vi "AI_ConfigurationRLC.vi"(8 "Error in":errorcluster, 10 "DAQ parameters":T1={"Trigger level"=1.0204081632653061, "Trigger slope"=10280, "Sampling rate (Hz)"=10000.0, "Number of sampes"=1000} {"Trigger slope" items=["Rising"=10280, "Falling"=10171]; "Trigger level" scale=0.0..10.0 scale format="%#_3g"}, 11 "Channels":T2) -> (0 "Error out":errorcluster, 3 "Task out":refnum<k21>)   [LabVIEW 2021]
uses:
  DAQmx_Channels.ctl
  DAQmx_Parameters.ctl
  <vilib>/DAQmx/create/channels.llb/DAQmx Create Channel (AI-Voltage-Basic).vi
  <vilib>/DAQmx/configure/timing.llb/DAQmx Timing (Sample Clock).vi
  <vilib>/DAQmx/configure/trigger.llb/DAQmx Start Trigger (Analog Edge).vi
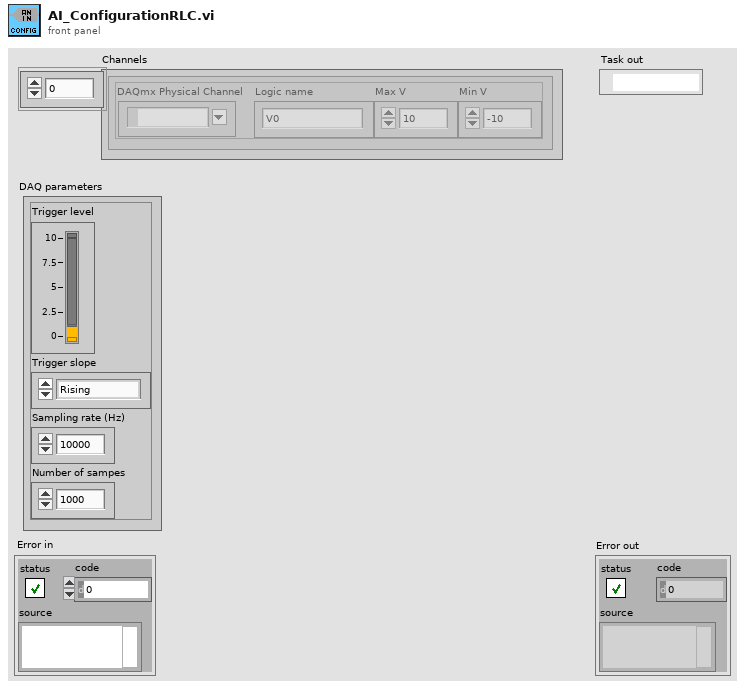
[diagram p1: front panel]
types:
  T1 = typedef "DAQmx_Parameters.ctl" = cluster{"Trigger level":dbl, "Trigger slope":u16, "Sampling rate (Hz)":dbl, "Number of sampes":i32}
  T2 = typedef "DAQmx_Channels.ctl" = cluster{"DAQmx Physical Channel":tag, "Logic name":string, "Max V":dbl, "Min V":dbl}[]
  T3 = cluster{"DAQmx Physical Channel":tag, "Logic name":string, "Max V":dbl, "Min V":dbl}
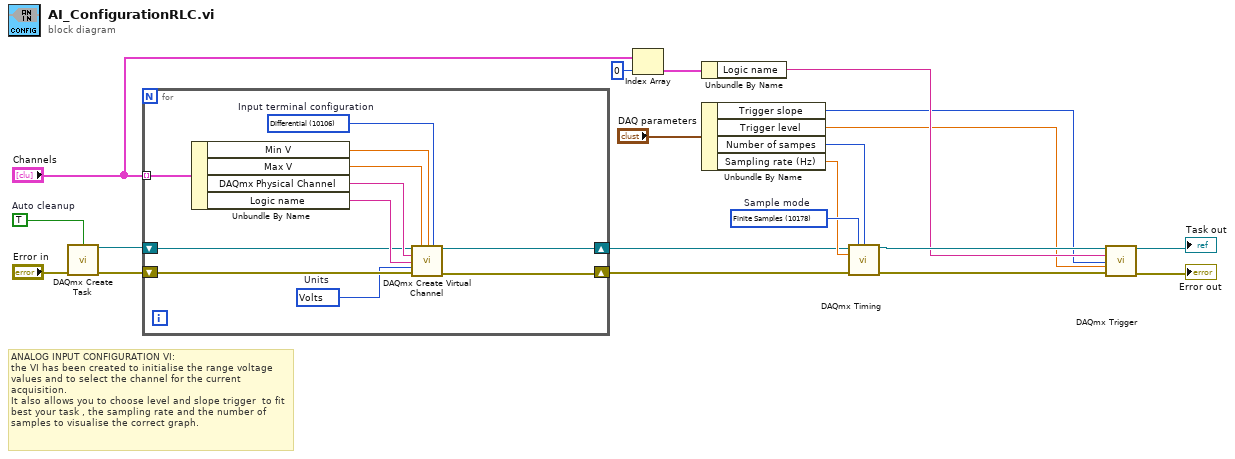
[diagram p0: block diagram]
diagram:
  w6 = TRUE  # Auto cleanup
  w17 = 10178 items=["Finite Samples"=10178, "Continuous Samples"=10123, "Hardware Timed Single Point"=12522]  # Sample mode
  # "ANALOG INPUT CONFIGURATION VI:\nthe VI has been created to initialise the range voltage values and to select the channel for the current acquisition. \nIt also allows you to choose level and slope trigger  to fit best your task , the sampling rate and the number of samples to visualise the correct graph."
  n1 = call <vilib>:"DAQmx Create Task.vi"("auto cleanup"=w6, "error in"="Error in") -> ("task out"=w20:refnum<k21>, "error out"=w19:errorcluster)  [unwired: 12 in]
  n2 = for {
    shift-right: [w29] -> w7
    shift-left: w20 -> [w21]
    shift-right: [w30] -> w18
    shift-left: w19 -> [w31]
    tunnel: "Channels" -> [w28] mode=indexing
    w22 = 10348 items=["Volts"=10348, "From Custom Scale"=10065]  # Units
    w23 = 10106 items=["Default"=-1, "RSE"=10083, "NRSE"=10078, "Differential"=10106, "Pseudodifferential"=12529]  # Input terminal configuration
    n3 = Unbundle By Name(w28) -> ("Min V"=w27:dbl, "Max V"=w24:dbl, "DAQmx Physical Channel"=w26:tag, "Logic name"=w25:string)
    n4 = call-poly <vilib>:"DAQmx Create Virtual Channel.vi"("task in"=w21, "maximum value"=w24, "minimum value"=w27, "input terminal configuration"=w23, "physical channels"=w26, "name to assign"=w25, "units"=w22, "error in"=w31) -> ("task out"=w29:refnum<k21>, "error out"=w30:errorcluster)  [unwired: 6 in]
  }
  n5 = Index Array(array="Channels", index=0) -> (element=w11:T3)
  n6 = Unbundle By Name(w11) -> ("Logic name"=w5:string)
  n7 = Unbundle By Name("DAQ parameters") -> ("Trigger slope"=w2:u16, "Trigger level"=w1:dbl, "Number of sampes"=w15:i32, "Sampling rate (Hz)"=w14:dbl)
  n8 = call-poly <vilib>:"DAQmx Timing.vi"("task/channels in"=w7, "sample mode"=w17, "samples per channel"=w15, "rate"=w14, "error in"=w18) -> ("task out"=w13:refnum<k21>, "error out"=w12:errorcluster)  [unwired: 9 in]
  n9 = call-poly <vilib>:"DAQmx Trigger.vi"("task/channels in"=w13, "source"=w5, "slope"=w2, "level"=w1, "error in"=w12) -> ("task out"=→"Task out":refnum<k21>, "error out"=→"Error out":errorcluster)  [unwired: 9 in]
